vi "Read Write App Config.vi"(7 "Write (F)":bool, 8 "Error IN":errorcluster, 10 "App Config IN":T1={"Location"="", "Profiles Path"=path "", "Current Profile"="", "CA Number"="", "Cycles Completed"=0, "PWM Freq (Hz)"=0.0, "Controller Type:"=enum."Kuhnke", "Inform"="", "Pumps Present"=0, "Stagger Time (ms)"=0, "Tank 1 Fuel"="", "Tank 2 Fuel"="", "Serial Numbers"={"Position 1 SN"="", "Position 2 SN"="", "Poaition 3 SN"="", "Position 4 SN"="", "Position 5 SN"="", "Position 6 SN"=""}, "Constant Data Log"=FALSE, "VoltCtrlRef"="", "TenHzFrequency"=0, "VoltageSelect"=FALSE, "Watlow Present"=FALSE, "Temp 1"=0.0, "Temp 2"=0.0, "V_Run PI?"=FALSE, "Voltage Limits"={"V_Step"=1e-05, "V_CmdMax"=0.0, "V_CmdMin"=0.0}, "Voltage Far PI"={"V_FarSlew"=10.0, "V_FarKp"=0.0, "V_FarKi"=0.0}, "Voltage Mid PI"={"V_MidSlew"=10.0, "V_MidKp"=0.0, "V_MidKi"=0.0}, "Voltage Close PI"={"V_CloseSlew"=10.0, "V_CloseKp"=0.0, "V_CloseKi"=0.0}, "Voltage Scale"={"V_FFm"=0.0, "V_FFb"=0.0}, "Voltage Cutoffs"={"V_MidCutoff"=0.0, "V_CloseCutoff"=0.0}, "Pressure Scale"={"Pres_FFm"=1e-05, "Pres_FFb"=0.0}, "Temp Format"=0, "Temp Tolerance"=0.0}, 11 "Refnum in":T3) -> (0 "Error OUT":errorcluster, 2 "App Config OUT":T1={"Location"="", "Profiles Path"=path "", "Current Profile"="", "CA Number"="", "Cycles Completed"=0, "PWM Freq (Hz)"=0.0, "Controller Type:"=enum."Kuhnke", "Inform"="", "Pumps Present"=0, "Stagger Time (ms)"=0, "Tank 1 Fuel"="", "Tank 2 Fuel"="", "Serial Numbers"={"Position 1 SN"="", "Position 2 SN"="", "Poaition 3 SN"="", "Position 4 SN"="", "Position 5 SN"="", "Position 6 SN"=""}, "Constant Data Log"=FALSE, "VoltCtrlRef"="", "TenHzFrequency"=0, "VoltageSelect"=FALSE, "Watlow Present"=FALSE, "Temp 1"=0.0, "Temp 2"=0.0, "V_Run PI?"=FALSE, "Voltage Limits"={"V_Step"=1e-05, "V_CmdMax"=0.0, "V_CmdMin"=0.0}, "Voltage Far PI"={"V_FarSlew"=10.0, "V_FarKp"=0.0, "V_FarKi"=0.0}, "Voltage Mid PI"={"V_MidSlew"=10.0, "V_MidKp"=0.0, "V_MidKi"=0.0}, "Voltage Close PI"={"V_CloseSlew"=10.0, "V_CloseKp"=0.0, "V_CloseKi"=0.0}, "Voltage Scale"={"V_FFm"=0.0, "V_FFb"=0.0}, "Voltage Cutoffs"={"V_MidCutoff"=0.0, "V_CloseCutoff"=0.0}, "Pressure Scale"={"Pres_FFm"=1e-05, "Pres_FFb"=0.0}, "Temp Format"=0, "Temp Tolerance"=0.0}, 3 "Refnum out":T3)   [LabVIEW 2013]
uses:
  <vilib>/Utility/config.llb/Config Data RefNum.ctl
  Type Defs/App Config.ctl
  Type Defs/Controller Names.ctl
  <vilib>/Utility/config.llb/Write Key (String).vi
  <vilib>/Utility/config.llb/Write Key (Path).vi
  <vilib>/Utility/config.llb/Write Key (U32).vi
  <vilib>/Utility/config.llb/Write Key (Double).vi
  <vilib>/Utility/config.llb/Write Key (I32).vi
  <vilib>/Utility/config.llb/Write Key (Boolean).vi
  <vilib>/Utility/config.llb/Read Key (String).vi
  <vilib>/Utility/config.llb/Read Key (Path).vi
  <vilib>/Utility/config.llb/Read Key (U32).vi
  <vilib>/Utility/config.llb/Read Key (Double).vi
  <vilib>/Utility/config.llb/Read Key (I32).vi
  <vilib>/Utility/config.llb/Read Key (Boolean).vi
  <vilib>/Utility/config.llb/NI_LVConfig.lvlib
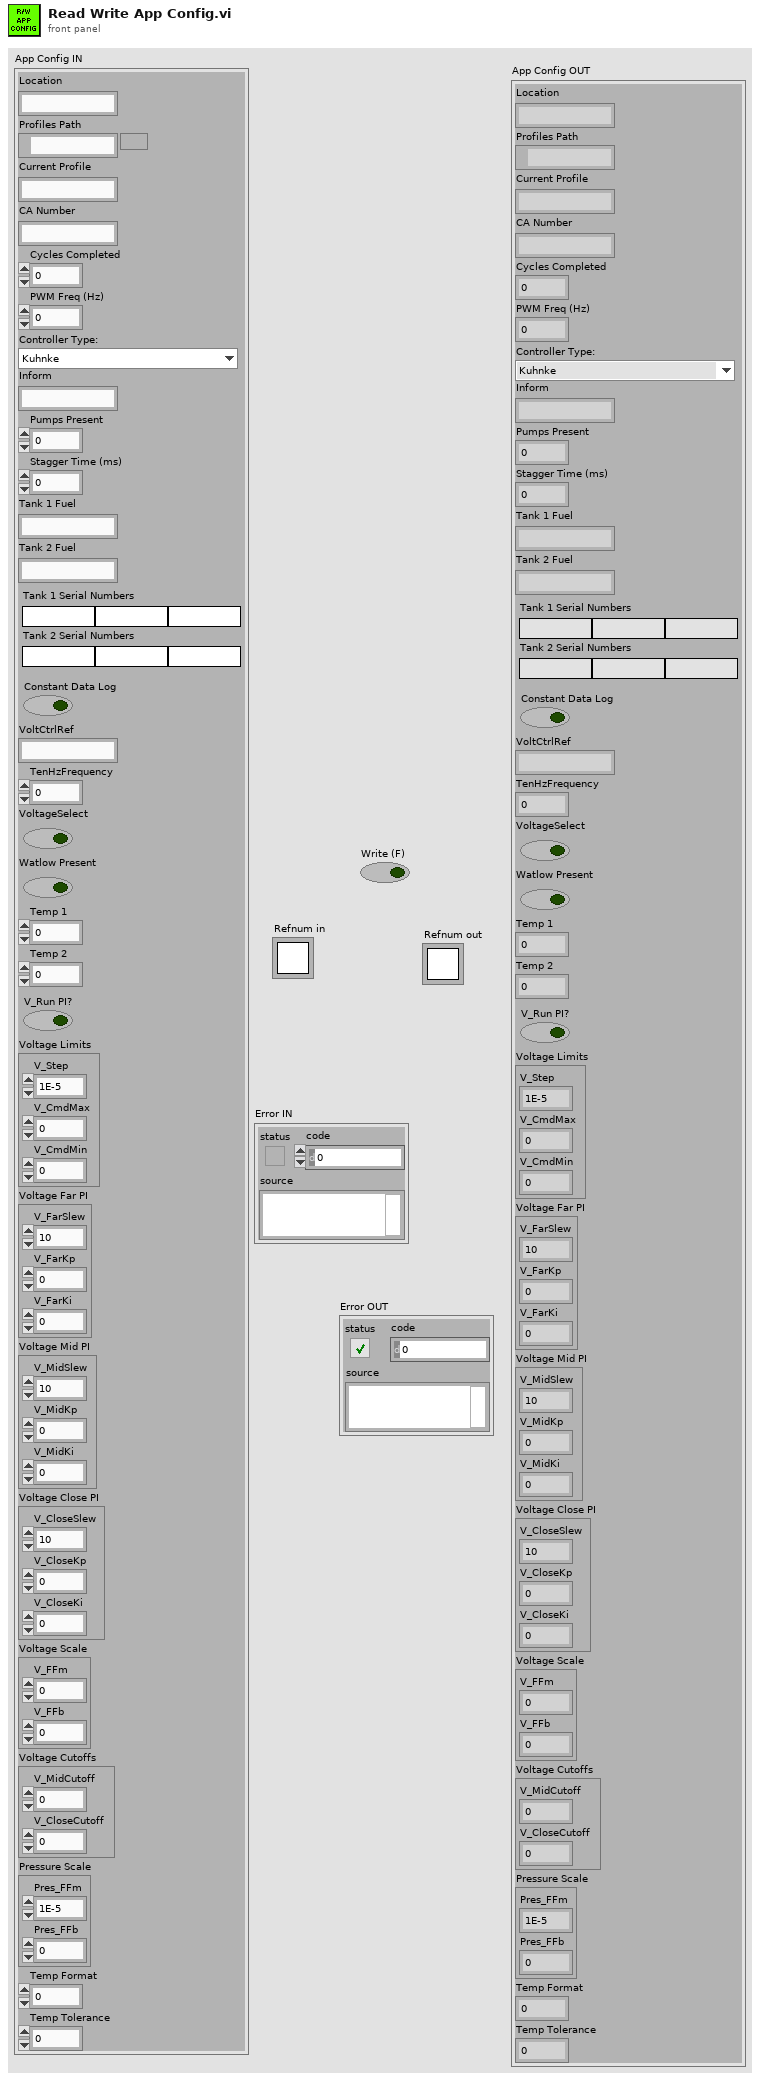
[diagram p1: front panel]
types:
  T1 = typedef "App Config.ctl" = cluster{"Location":string, "Profiles Path":path, "Current Profile":string, "CA Number":string, "Cycles Completed":u32, "PWM Freq (Hz)":dbl, "Controller Type:":T2, "Inform":string, "Pumps Present":u32, "Stagger Time (ms)":i32, "Tank 1 Fuel":string, "Tank 2 Fuel":string, "Serial Numbers":cluster{"Position 1 SN":string, "Position 2 SN":string, "Poaition 3 SN":string, "Position 4 SN":string, "Position 5 SN":string, "Position 6 SN":string}, "Constant Data Log":bool, "VoltCtrlRef":string, "TenHzFrequency":u32, "VoltageSelect":bool, "Watlow Present":bool, "Temp 1":dbl, "Temp 2":dbl, "V_Run PI?":bool, "Voltage Limits":cluster{"V_Step":dbl, "V_CmdMax":dbl, "V_CmdMin":dbl}, "Voltage Far PI":cluster{"V_FarSlew":dbl, "V_FarKp":dbl, "V_FarKi":dbl}, "Voltage Mid PI":cluster{"V_MidSlew":dbl, "V_MidKp":dbl, "V_MidKi":dbl}, "Voltage Close PI":cluster{"V_CloseSlew":dbl, "V_CloseKp":dbl, "V_CloseKi":dbl}, "Voltage Scale":cluster{"V_FFm":dbl, "V_FFb":dbl}, "Voltage Cutoffs":cluster{"V_MidCutoff":dbl, "V_CloseCutoff":dbl}, "Pressure Scale":cluster{"Pres_FFm":dbl, "Pres_FFb":dbl}, "Temp Format":i32, "Temp Tolerance":dbl}
  T2 = typedef "Controller Names.ctl" = enum16{"Kuhnke", "Helbako BLDC", "Conti", "Hella BLDC OL PWM", "Hella BLDC Turbine OL PWM", "Helbako (old)", "TI PWM", "PSA", "Hella Gas", "Hella Diesel", "8 Comm", "10 Comm", "8 Comm Hella", "10 Comm Hella", "8 Comm Omron", "10 Comm Omron", "8 Comm Nissan", "10 Comm Nissan"}
  T3 = typedef "NI_LVConfig.lvlib/Config Data RefNum.ctl" = refnum<k1>
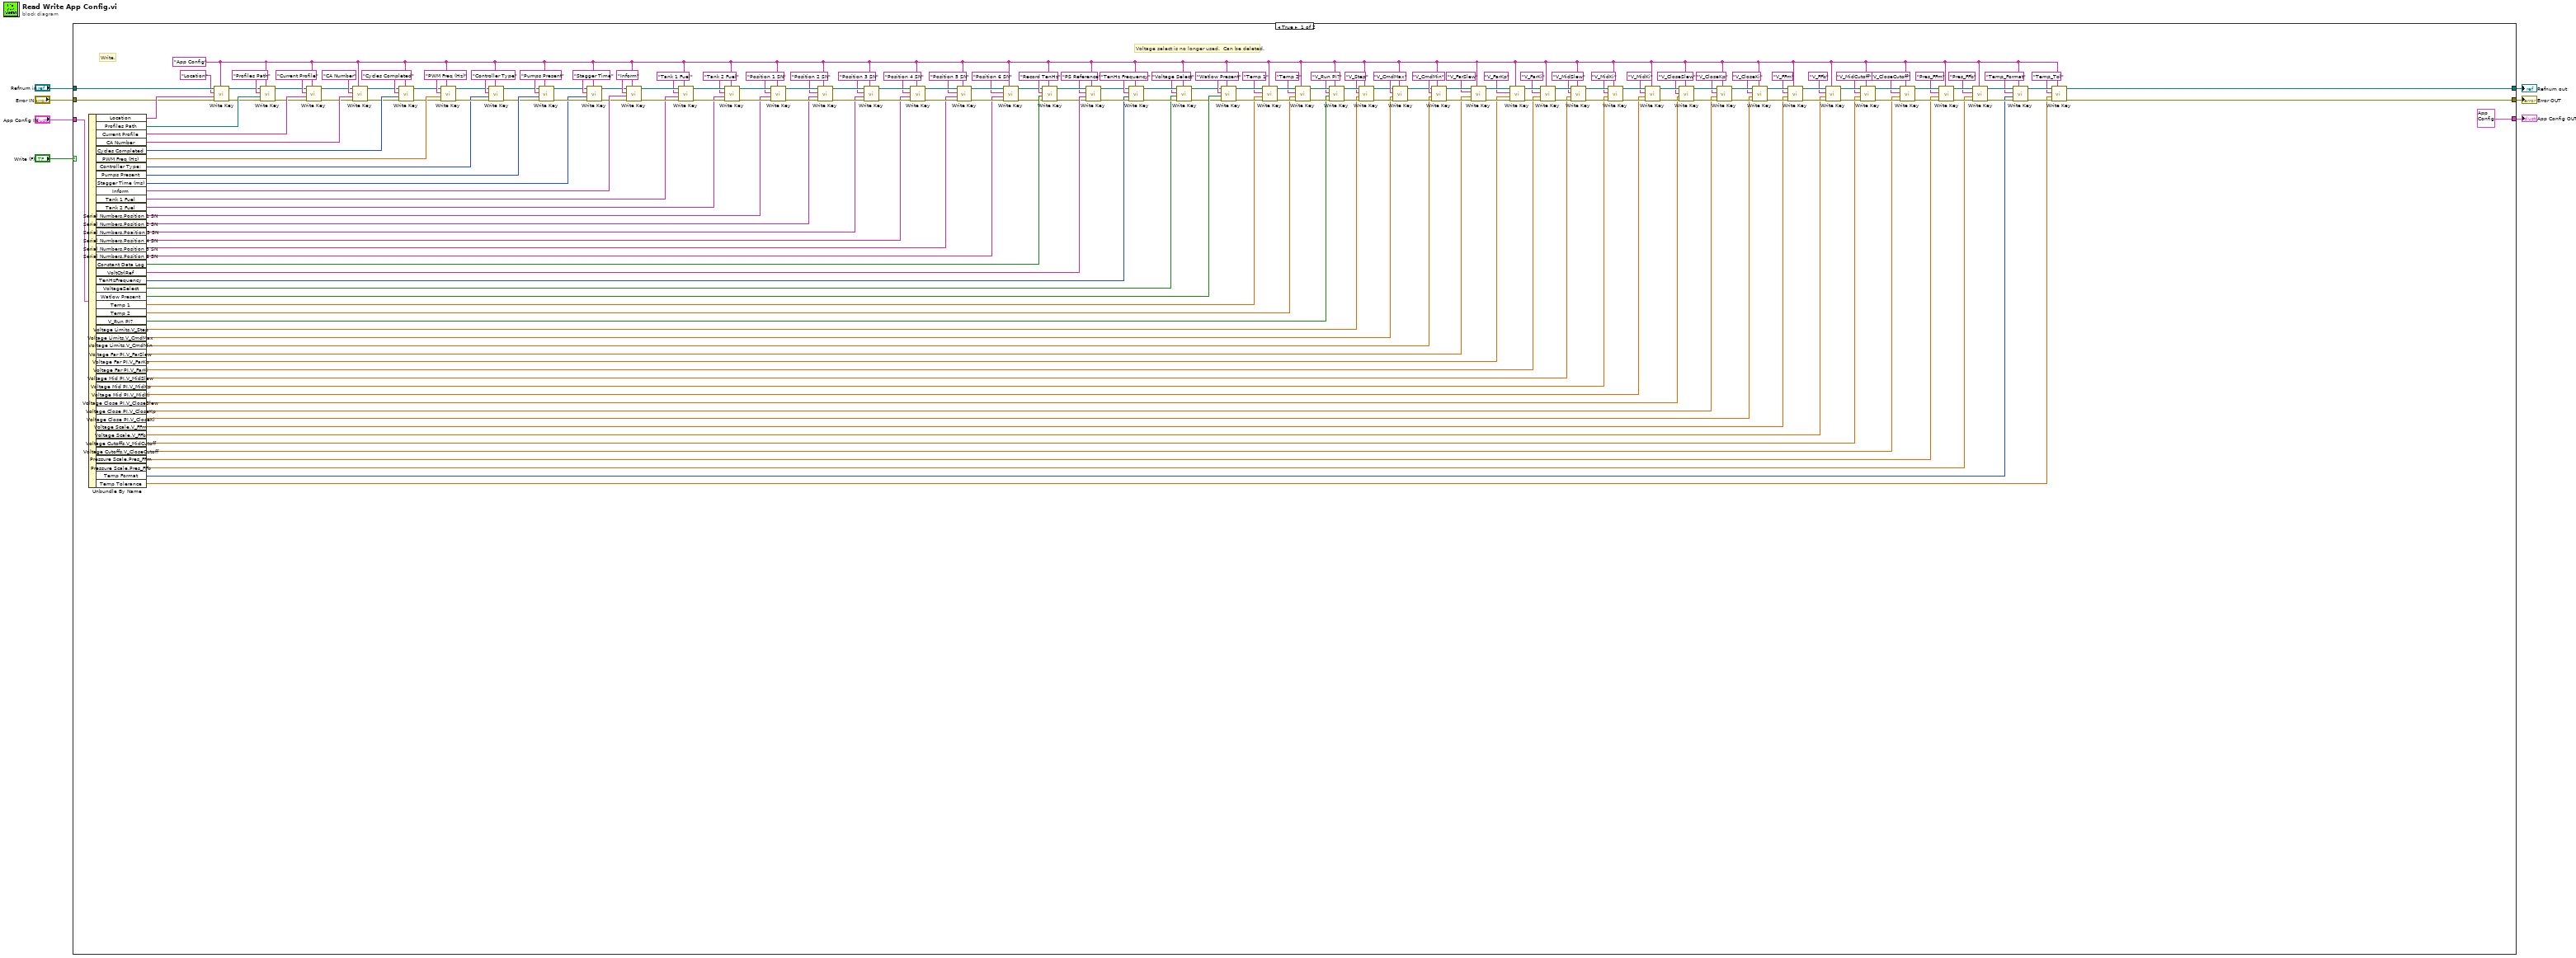
[diagram p0: block diagram]
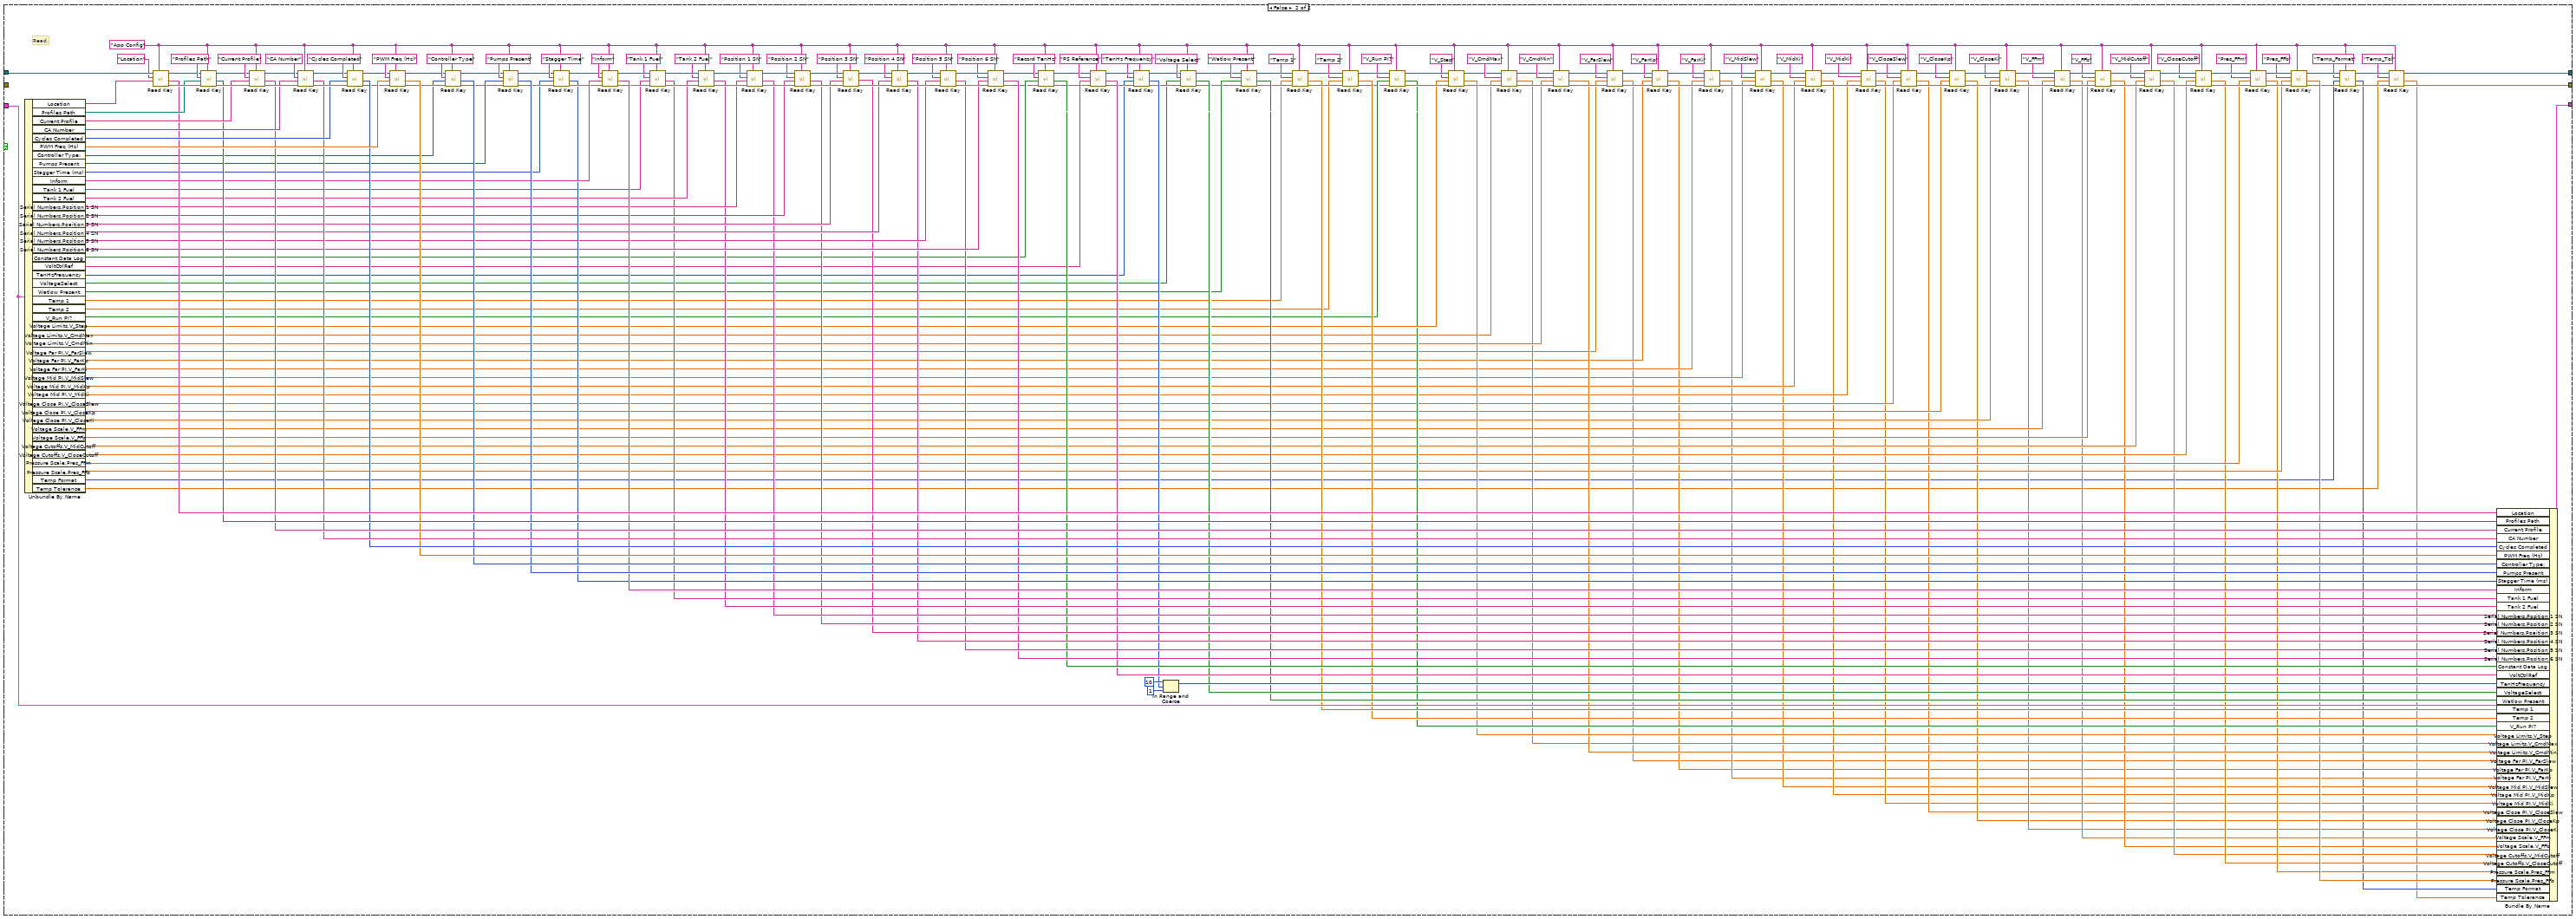
[diagram p2: hidden frame]
diagram:
  n1 = case shown="True" "Write (F)" {
    tunnel: "App Config IN" -> [w196 w385]
    tunnel: "Refnum in" -> [w195 w433]
    tunnel: [w13 w204] -> w4
    tunnel: [w14 w203] -> w3
    tunnel: [T1 {"Location"="", "Profiles Path"=path "", "Current Profile"="", "CA Number"="", "Cycles Completed"=0, "PWM Freq (Hz)"=0.0, "Controller Type:"=enum."Kuhnke", "Inform"="", "Pumps Present"=0, "Stagger Time (ms)"=0, "Tank 1 Fuel"="", "Tank 2 Fuel"="", "Serial Numbers"={"Position 1 SN"="", "Position 2 SN"="", "Poaition 3 SN"="", "Position 4 SN"="", "Position 5 SN"="", "Position 6 SN"=""}, "Constant Data Log"=FALSE, "VoltCtrlRef"="", "TenHzFrequency"=0, "VoltageSelect"=FALSE, "Watlow Present"=FALSE, "Temp 1"=0.0, "Temp 2"=0.0, "V_Run PI?"=FALSE, "Voltage Limits"={"V_Step"=0.0, "V_CmdMax"=0.0, "V_CmdMin"=0.0}, "Voltage Far PI"={"V_FarSlew"=0.0, "V_FarKp"=0.0, "V_FarKi"=0.0}, "Voltage Mid PI"={"V_MidSlew"=0.0, "V_MidKp"=0.0, "V_MidKi"=0.0}, "Voltage Close PI"={"V_CloseSlew"=0.0, "V_CloseKp"=0.0, "V_CloseKi"=0.0}, "Voltage Scale"={"V_FFm"=0.0, "V_FFb"=0.0}, "Voltage Cutoffs"={"V_MidCutoff"=0.0, "V_CloseCutoff"=0.0}, "Pressure Scale"={"Pres_FFm"=0.0, "Pres_FFb"=0.0}, "Temp Format"=0, "Temp Tolerance"=0.0} ("App Config IN") w384] -> w2
    tunnel: "Error IN" -> [w173 _]
    frame True {
      w12 = "App Config" ("section")
      # "Voltage select is no longer used.  Can be deleted."
      # "Write."
      n2 = Unbundle By Name(w196) -> ("Location"=w193:string, "Profiles Path"=w187:path, "Current Profile"=w186:string, "CA Number"=w185:string, "Cycles Completed"=w184:u32, "PWM Freq (Hz)"=w183:dbl, "Controller Type:"=w170:T2, "Pumps Present"=w165:u32, "Stagger Time (ms)"=w155:i32, "Inform"=w161:string, "Tank 1 Fuel"=w138:string, "Tank 2 Fuel"=w137:string, "Serial Numbers.Position 1 SN"=w136:string, "Serial Numbers.Position 2 SN"=w135:string, "Serial Numbers.Poaition 3 SN"=w134:string, "Serial Numbers.Position 4 SN"=w133:string, "Serial Numbers.Position 5 SN"=w132:string, "Serial Numbers.Position 6 SN"=w131:string, "Constant Data Log"=w121:bool, "VoltCtrlRef"=w120:string, "TenHzFrequency"=w113:u32, "VoltageSelect"=w107:bool, "Watlow Present"=w105:bool, "Temp 1"=w95:dbl, "Temp 2"=w96:dbl, "V_Run PI?"=w90:bool, "Voltage Limits.V_Step"=w89:dbl, "Voltage Limits.V_CmdMax"=w72:dbl, "Voltage Limits.V_CmdMin"=w71:dbl, "Voltage Far PI.V_FarSlew"=w33:dbl, "Voltage Far PI.V_FarKp"=w32:dbl, "Voltage Far PI.V_FarKi"=w31:dbl, "Voltage Mid PI.V_MidSlew"=w30:dbl, "Voltage Mid PI.V_MidKp"=w29:dbl, "Voltage Mid PI.V_MidKi"=w28:dbl, "Voltage Close PI.V_CloseSlew"=w27:dbl, "Voltage Close PI.V_CloseKp"=w26:dbl, "Voltage Close PI.V_CloseKi"=w25:dbl, "Voltage Scale.V_FFm"=w24:dbl, "Voltage Scale.V_FFb"=w23:dbl, "Voltage Cutoffs.V_MidCutoff"=w22:dbl, "Voltage Cutoffs.V_CloseCutoff"=w21:dbl, "Pressure Scale.Pres_FFm"=w20:dbl, "Pressure Scale.Pres_FFb"=w19:dbl, "Temp Format"=w9:i32, "Temp Tolerance"=w8:dbl)
      n3 = call-poly <vilib>:"Write Key.vi"("section"=w12, "error in (no error)"=w173, "value"=w193, "key"="Location" ("section"), "refnum"=w195) -> ("error out"=w182:errorcluster, "refnum out"=w181:T3)  [unwired: 4 in, 1 out]
      n4 = call-poly <vilib>:"Write Key.vi"("section"=w12, "error in (no error)"=w182, "value"=w187, "key"="Profiles Path" ("section"), "refnum"=w181) -> ("error out"=w179:errorcluster, "refnum out"=w180:T3)  [unwired: 4 in, 1 out]
      n5 = call-poly <vilib>:"Write Key.vi"("section"=w12, "error in (no error)"=w179, "value"=w186, "key"="Current Profile" ("section"), "refnum"=w180) -> ("error out"=w177:errorcluster, "refnum out"=w178:T3)  [unwired: 4 in, 1 out]
      n6 = call-poly <vilib>:"Write Key.vi"("section"=w12, "error in (no error)"=w177, "value"=w185, "key"="CA Number" ("section"), "refnum"=w178) -> ("error out"=w175:errorcluster, "refnum out"=w176:T3)  [unwired: 4 in, 1 out]
      n7 = call-poly <vilib>:"Write Key.vi"("section"=w12, "error in (no error)"=w175, "value"=w184, "key"="Cycles Completed" ("section"), "refnum"=w176) -> ("error out"=w167:errorcluster, "refnum out"=w168:T3)  [unwired: 4 in, 1 out]
      n8 = call-poly <vilib>:"Write Key.vi"("section"=w12, "error in (no error)"=w167, "value"=w183, "key"="PWM Freq (Hz)" ("section"), "refnum"=w168) -> ("error out"=w171:errorcluster, "refnum out"=w169:T3)  [unwired: 4 in, 1 out]
      n9 = call-poly <vilib>:"Write Key.vi"("section"=w12, "error in (no error)"=w171, "value"=w170, "key"="Controller Type" ("section"), "refnum"=w169) -> ("error out"=w163:errorcluster, "refnum out"=w164:T3)  [unwired: 4 in, 1 out]
      n10 = call-poly <vilib>:"Write Key.vi"("section"=w12, "error in (no error)"=w163, "value"=w165, "key"="Pumps Present" ("section"), "refnum"=w164) -> ("error out"=w158:errorcluster, "refnum out"=w159:T3)  [unwired: 4 in, 1 out]
      n11 = call-poly <vilib>:"Write Key.vi"("section"=w12, "error in (no error)"=w158, "value"=w155, "key"="Stagger Time" ("section"), "refnum"=w159) -> ("error out"=w157:errorcluster, "refnum out"=w156:T3)  [unwired: 4 in, 1 out]
      n12 = call-poly <vilib>:"Write Key.vi"("section"=w12, "error in (no error)"=w157, "value"=w161, "key"="Inform" ("section"), "refnum"=w156) -> ("error out"=w139:errorcluster, "refnum out"=w154:T3)  [unwired: 4 in, 1 out]
      n13 = call-poly <vilib>:"Write Key.vi"("section"=w12, "error in (no error)"=w139, "value"=w138, "key"="Tank 1 Fuel", "refnum"=w154) -> ("error out"=w140:errorcluster, "refnum out"=w153:T3)  [unwired: 4 in, 1 out]
      n14 = call-poly <vilib>:"Write Key.vi"("section"=w12, "error in (no error)"=w140, "value"=w137, "key"="Tank 2 Fuel", "refnum"=w153) -> ("error out"=w141:errorcluster, "refnum out"=w152:T3)  [unwired: 4 in, 1 out]
      n15 = call-poly <vilib>:"Write Key.vi"("section"=w12, "error in (no error)"=w141, "value"=w136, "key"="Position 1 SN", "refnum"=w152) -> ("error out"=w142:errorcluster, "refnum out"=w151:T3)  [unwired: 4 in, 1 out]
      n16 = call-poly <vilib>:"Write Key.vi"("section"=w12, "error in (no error)"=w142, "value"=w135, "key"="Position 2 SN", "refnum"=w151) -> ("error out"=w143:errorcluster, "refnum out"=w150:T3)  [unwired: 4 in, 1 out]
      n17 = call-poly <vilib>:"Write Key.vi"("section"=w12, "error in (no error)"=w143, "value"=w134, "key"="Position 3 SN", "refnum"=w150) -> ("error out"=w144:errorcluster, "refnum out"=w149:T3)  [unwired: 4 in, 1 out]
      n18 = call-poly <vilib>:"Write Key.vi"("section"=w12, "error in (no error)"=w144, "value"=w133, "key"="Position 4 SN", "refnum"=w149) -> ("error out"=w145:errorcluster, "refnum out"=w148:T3)  [unwired: 4 in, 1 out]
      n19 = call-poly <vilib>:"Write Key.vi"("section"=w12, "error in (no error)"=w145, "value"=w132, "key"="Position 5 SN", "refnum"=w148) -> ("error out"=w146:errorcluster, "refnum out"=w147:T3)  [unwired: 4 in, 1 out]
      n20 = call-poly <vilib>:"Write Key.vi"("section"=w12, "error in (no error)"=w146, "value"=w131, "key"="Position 6 SN", "refnum"=w147) -> ("error out"=w111:errorcluster, "refnum out"=w112:T3)  [unwired: 4 in, 1 out]
      n21 = call-poly <vilib>:"Write Key.vi"("section"=w12, "error in (no error)"=w111, "value"=w121, "key"="Record TenHz", "refnum"=w112) -> ("error out"=w119:errorcluster, "refnum out"=w118:T3)  [unwired: 4 in, 1 out]
      n22 = call-poly <vilib>:"Write Key.vi"("section"=w12, "error in (no error)"=w119, "value"=w120, "key"="PS Reference", "refnum"=w118) -> ("error out"=w115:errorcluster, "refnum out"=w114:T3)  [unwired: 4 in, 1 out]
      n23 = call-poly <vilib>:"Write Key.vi"("section"=w12, "error in (no error)"=w115, "value"=w113, "key"="TenHz Frequency", "refnum"=w114) -> ("error out"=w109:errorcluster, "refnum out"=w110:T3)  [unwired: 4 in, 1 out]
      n24 = call-poly <vilib>:"Write Key.vi"("section"=w12, "error in (no error)"=w109, "value"=w107, "key"="Voltage Select", "refnum"=w110) -> ("error out"=w103:errorcluster, "refnum out"=w104:T3)  [unwired: 4 in, 1 out]
      n25 = call-poly <vilib>:"Write Key.vi"("section"=w12, "error in (no error)"=w103, "value"=w105, "key"="Watlow Present", "refnum"=w104) -> ("error out"=w100:errorcluster, "refnum out"=w102:T3)  [unwired: 4 in, 1 out]
      n26 = call-poly <vilib>:"Write Key.vi"("section"=w12, "error in (no error)"=w100, "value"=w95, "key"="Temp 1", "refnum"=w102) -> ("error out"=w99:errorcluster, "refnum out"=w101:T3)  [unwired: 4 in, 1 out]
      n27 = call-poly <vilib>:"Write Key.vi"("section"=w12, "error in (no error)"=w99, "value"=w96, "key"="Temp 2", "refnum"=w101) -> ("error out"=w92:errorcluster, "refnum out"=w93:T3)  [unwired: 4 in, 1 out]
      n28 = call-poly <vilib>:"Write Key.vi"("section"=w12, "error in (no error)"=w92, "value"=w90, "key"="V_Run PI?" ("section"), "refnum"=w93) -> ("error out"=w91:errorcluster, "refnum out"=w94:T3)  [unwired: 4 in, 1 out]
      n29 = call-poly <vilib>:"Write Key.vi"("section"=w12, "error in (no error)"=w91, "value"=w89, "key"="V_Step" ("section"), "refnum"=w94) -> ("error out"=w84:errorcluster, "refnum out"=w78:T3)  [unwired: 4 in, 1 out]
      n30 = call-poly <vilib>:"Write Key.vi"("section"=w12, "error in (no error)"=w84, "value"=w72, "key"="V_CmdMax" ("section"), "refnum"=w78) -> ("error out"=w83:errorcluster, "refnum out"=w77:T3)  [unwired: 4 in, 1 out]
      n31 = call-poly <vilib>:"Write Key.vi"("section"=w12, "error in (no error)"=w83, "value"=w71, "key"="V_CmdMin" ("section"), "refnum"=w77) -> ("error out"=w57:errorcluster, "refnum out"=w66:T3)  [unwired: 4 in, 1 out]
      n32 = call-poly <vilib>:"Write Key.vi"("section"=w12, "error in (no error)"=w57, "value"=w33, "key"="V_FarSlew", "refnum"=w66) -> ("error out"=w58:errorcluster, "refnum out"=w65:T3)  [unwired: 4 in, 1 out]
      n33 = call-poly <vilib>:"Write Key.vi"("section"=w12, "error in (no error)"=w58, "value"=w32, "key"="V_FarKp", "refnum"=w65) -> ("error out"=w59:errorcluster, "refnum out"=w64:T3)  [unwired: 4 in, 1 out]
      n34 = call-poly <vilib>:"Write Key.vi"("section"=w12, "error in (no error)"=w59, "value"=w31, "key"="V_FarKi", "refnum"=w64) -> ("error out"=w60:errorcluster, "refnum out"=w63:T3)  [unwired: 4 in, 1 out]
      n35 = call-poly <vilib>:"Write Key.vi"("section"=w12, "error in (no error)"=w60, "value"=w30, "key"="V_MidSlew", "refnum"=w63) -> ("error out"=w61:errorcluster, "refnum out"=w62:T3)  [unwired: 4 in, 1 out]
      n36 = call-poly <vilib>:"Write Key.vi"("section"=w12, "error in (no error)"=w61, "value"=w29, "key"="V_MidKi", "refnum"=w62) -> ("error out"=w82:errorcluster, "refnum out"=w76:T3)  [unwired: 4 in, 1 out]
      n37 = call-poly <vilib>:"Write Key.vi"("section"=w12, "error in (no error)"=w82, "value"=w28, "key"="V_MidKi", "refnum"=w76) -> ("error out"=w81:errorcluster, "refnum out"=w75:T3)  [unwired: 4 in, 1 out]
      n38 = call-poly <vilib>:"Write Key.vi"("section"=w12, "error in (no error)"=w81, "value"=w27, "key"="V_CloseSlew", "refnum"=w75) -> ("error out"=w80:errorcluster, "refnum out"=w74:T3)  [unwired: 4 in, 1 out]
      n39 = call-poly <vilib>:"Write Key.vi"("section"=w12, "error in (no error)"=w80, "value"=w26, "key"="V_CloseKp", "refnum"=w74) -> ("error out"=w79:errorcluster, "refnum out"=w73:T3)  [unwired: 4 in, 1 out]
      n40 = call-poly <vilib>:"Write Key.vi"("section"=w12, "error in (no error)"=w79, "value"=w25, "key"="V_CloseKi", "refnum"=w73) -> ("error out"=w67:errorcluster, "refnum out"=w70:T3)  [unwired: 4 in, 1 out]
      n41 = call-poly <vilib>:"Write Key.vi"("section"=w12, "error in (no error)"=w67, "value"=w24, "key"="V_FFm", "refnum"=w70) -> ("error out"=w68:errorcluster, "refnum out"=w69:T3)  [unwired: 4 in, 1 out]
      n42 = call-poly <vilib>:"Write Key.vi"("section"=w12, "error in (no error)"=w68, "value"=w23, "key"="V_FFb", "refnum"=w69) -> ("error out"=w49:errorcluster, "refnum out"=w53:T3)  [unwired: 4 in, 1 out]
      n43 = call-poly <vilib>:"Write Key.vi"("section"=w12, "error in (no error)"=w49, "value"=w22, "key"="V_MidCutoff", "refnum"=w53) -> ("error out"=w50:errorcluster, "refnum out"=w54:T3)  [unwired: 4 in, 1 out]
      n44 = call-poly <vilib>:"Write Key.vi"("section"=w12, "error in (no error)"=w50, "value"=w21, "key"="V_CloseCutoff", "refnum"=w54) -> ("error out"=w51:errorcluster, "refnum out"=w55:T3)  [unwired: 4 in, 1 out]
      n45 = call-poly <vilib>:"Write Key.vi"("section"=w12, "error in (no error)"=w51, "value"=w20, "key"="Pres_FFm", "refnum"=w55) -> ("error out"=w52:errorcluster, "refnum out"=w56:T3)  [unwired: 4 in, 1 out]
      n46 = call-poly <vilib>:"Write Key.vi"("section"=w12, "error in (no error)"=w52, "value"=w19, "key"="Pres_FFb", "refnum"=w56) -> ("error out"=w15:errorcluster, "refnum out"=w18:T3)  [unwired: 4 in, 1 out]
      n47 = call-poly <vilib>:"Write Key.vi"("section"=w12, "error in (no error)"=w15, "value"=w9, "key"="Temp_Format", "refnum"=w18) -> ("error out"=w16:errorcluster, "refnum out"=w17:T3)  [unwired: 4 in, 1 out]
      n48 = call-poly <vilib>:"Write Key.vi"("section"=w12, "error in (no error)"=w16, "value"=w8, "key"="Temp_Tol", "refnum"=w17) -> ("error out"=w14:errorcluster, "refnum out"=w13:T3)  [unwired: 4 in, 1 out]
    }
    frame False {
      w209 = "App Config" ("section")
      # "Read."
      n49 = Unbundle By Name(w385) -> ("Location"=w418:string, "Profiles Path"=w417:path, "Current Profile"=w416:string, "CA Number"=w415:string, "Cycles Completed"=w414:u32, "PWM Freq (Hz)"=w413:dbl, "Controller Type:"=w331:T2, "Pumps Present"=w399:u32, "Stagger Time (ms)"=w387:i32, "Inform"=w394:string, "Tank 1 Fuel"=w359:string, "Tank 2 Fuel"=w358:string, "Serial Numbers.Position 1 SN"=w357:string, "Serial Numbers.Position 2 SN"=w356:string, "Serial Numbers.Poaition 3 SN"=w355:string, "Serial Numbers.Position 4 SN"=w354:string, "Serial Numbers.Position 5 SN"=w353:string, "Serial Numbers.Position 6 SN"=w352:string, "Constant Data Log"=w342:bool, "VoltCtrlRef"=w339:string, "TenHzFrequency"=w333:u32, "VoltageSelect"=w321:bool, "Watlow Present"=w318:bool, "Temp 1"=w306:dbl, "Temp 2"=w305:dbl, "V_Run PI?"=w302:bool, "Voltage Limits.V_Step"=w301:dbl, "Voltage Limits.V_CmdMax"=w278:dbl, "Voltage Limits.V_CmdMin"=w277:dbl, "Voltage Far PI.V_FarSlew"=w239:dbl, "Voltage Far PI.V_FarKp"=w238:dbl, "Voltage Far PI.V_FarKi"=w237:dbl, "Voltage Mid PI.V_MidSlew"=w236:dbl, "Voltage Mid PI.V_MidKp"=w235:dbl, "Voltage Mid PI.V_MidKi"=w234:dbl, "Voltage Close PI.V_CloseSlew"=w233:dbl, "Voltage Close PI.V_CloseKp"=w232:dbl, "Voltage Close PI.V_CloseKi"=w231:dbl, "Voltage Scale.V_FFm"=w230:dbl, "Voltage Scale.V_FFb"=w229:dbl, "Voltage Cutoffs.V_MidCutoff"=w228:dbl, "Voltage Cutoffs.V_CloseCutoff"=w227:dbl, "Pressure Scale.Pres_FFm"=w226:dbl, "Pressure Scale.Pres_FFb"=w225:dbl, "Temp Format"=w197:i32, "Temp Tolerance"=w198:dbl)
      n50 = call-poly <vilib>:"Read Key.vi"("section"=w209, "default value"=w418, "key"="Location" ("section"), "refnum"=w433) -> ("error out"=w426:errorcluster, "value"=w412:string, "refnum out"=w425:T3)  [unwired: 4 in, 1 out]
      n51 = call-poly <vilib>:"Read Key.vi"("section"=w209, "error in (no error)"=w426, "default value"=w417, "key"="Profiles Path" ("section"), "refnum"=w425) -> ("error out"=w423:errorcluster, "value"=w411:path, "refnum out"=w424:T3)  [unwired: 3 in, 1 out]
      n52 = call-poly <vilib>:"Read Key.vi"("section"=w209, "error in (no error)"=w423, "default value"=w416, "key"="Current Profile" ("section"), "refnum"=w424) -> ("error out"=w421:errorcluster, "value"=w410:string, "refnum out"=w422:T3)  [unwired: 3 in, 1 out]
      n53 = call-poly <vilib>:"Read Key.vi"("section"=w209, "error in (no error)"=w421, "default value"=w415, "key"="CA Number" ("section"), "refnum"=w422) -> ("error out"=w419:errorcluster, "value"=w409:string, "refnum out"=w420:T3)  [unwired: 3 in, 1 out]
      n54 = call-poly <vilib>:"Read Key.vi"("section"=w209, "error in (no error)"=w419, "default value"=w414, "key"="Cycles Completed" ("section"), "refnum"=w420) -> ("error out"=w401:errorcluster, "value"=w408:u32, "refnum out"=w402:T3)  [unwired: 3 in, 1 out]
      n55 = call-poly <vilib>:"Read Key.vi"("section"=w209, "error in (no error)"=w401, "default value"=w413, "key"="PWM Freq (Hz)" ("section"), "refnum"=w402) -> ("error out"=w404:errorcluster, "value"=w407:dbl, "refnum out"=w405:T3)  [unwired: 3 in, 1 out]
      n56 = call-poly <vilib>:"Read Key.vi"("section"=w209, "error in (no error)"=w404, "default value"=w331, "key"="Controller Type" ("section"), "refnum"=w405) -> ("error out"=w398:errorcluster, "value"=w403:i32, "refnum out"=w397:T3)  [unwired: 3 in, 1 out]
      n57 = call-poly <vilib>:"Read Key.vi"("section"=w209, "error in (no error)"=w398, "default value"=w399, "key"="Pumps Present" ("section"), "refnum"=w397) -> ("error out"=w391:errorcluster, "value"=w396:u32, "refnum out"=w390:T3)  [unwired: 3 in, 1 out]
      n58 = call-poly <vilib>:"Read Key.vi"("section"=w209, "error in (no error)"=w391, "default value"=w387, "key"="Stagger Time" ("section"), "refnum"=w390) -> ("error out"=w388:errorcluster, "value"=w386:i32, "refnum out"=w389:T3)  [unwired: 3 in, 1 out]
      n59 = call-poly <vilib>:"Read Key.vi"("section"=w209, "error in (no error)"=w388, "default value"=w394, "key"="Inform" ("section"), "refnum"=w389) -> ("error out"=w375:errorcluster, "value"=w393:string, "refnum out"=w383:T3)  [unwired: 3 in, 1 out]
      n60 = call-poly <vilib>:"Read Key.vi"("section"=w209, "error in (no error)"=w375, "default value"=w359, "key"="Tank 1 Fuel", "refnum"=w383) -> ("error out"=w374:errorcluster, "value"=w351:string, "refnum out"=w382:T3)  [unwired: 3 in, 1 out]
      n61 = call-poly <vilib>:"Read Key.vi"("section"=w209, "error in (no error)"=w374, "default value"=w358, "key"="Tank 2 Fuel", "refnum"=w382) -> ("error out"=w373:errorcluster, "value"=w350:string, "refnum out"=w381:T3)  [unwired: 3 in, 1 out]
      n62 = call-poly <vilib>:"Read Key.vi"("section"=w209, "error in (no error)"=w373, "default value"=w357, "key"="Position 1 SN", "refnum"=w381) -> ("error out"=w372:errorcluster, "value"=w349:string, "refnum out"=w380:T3)  [unwired: 3 in, 1 out]
      n63 = call-poly <vilib>:"Read Key.vi"("section"=w209, "error in (no error)"=w372, "default value"=w356, "key"="Position 2 SN", "refnum"=w380) -> ("error out"=w371:errorcluster, "value"=w348:string, "refnum out"=w379:T3)  [unwired: 3 in, 1 out]
      n64 = call-poly <vilib>:"Read Key.vi"("section"=w209, "error in (no error)"=w371, "default value"=w355, "key"="Position 3 SN", "refnum"=w379) -> ("error out"=w370:errorcluster, "value"=w347:string, "refnum out"=w378:T3)  [unwired: 3 in, 1 out]
      n65 = call-poly <vilib>:"Read Key.vi"("section"=w209, "error in (no error)"=w370, "default value"=w354, "key"="Position 4 SN", "refnum"=w378) -> ("error out"=w369:errorcluster, "value"=w346:string, "refnum out"=w377:T3)  [unwired: 3 in, 1 out]
      n66 = call-poly <vilib>:"Read Key.vi"("section"=w209, "error in (no error)"=w369, "default value"=w353, "key"="Position 5 SN", "refnum"=w377) -> ("error out"=w368:errorcluster, "value"=w345:string, "refnum out"=w376:T3)  [unwired: 3 in, 1 out]
      n67 = call-poly <vilib>:"Read Key.vi"("section"=w209, "error in (no error)"=w368, "default value"=w352, "key"="Position 6 SN", "refnum"=w376) -> ("error out"=w325:errorcluster, "value"=w344:string, "refnum out"=w326:T3)  [unwired: 3 in, 1 out]
      n68 = call-poly <vilib>:"Read Key.vi"("section"=w209, "error in (no error)"=w325, "default value"=w342, "key"="Record TenHz", "refnum"=w326) -> ("error out"=w338:errorcluster, "value"=w341:bool, "refnum out"=w337:T3)  [unwired: 3 in, 1 out]
      n69 = call-poly <vilib>:"Read Key.vi"("section"=w209, "error in (no error)"=w338, "default value"=w339, "key"="PS Reference", "refnum"=w337) -> ("error out"=w334:errorcluster, "value"=w336:string, "refnum out"=w335:T3)  [unwired: 3 in, 1 out]
      n70 = call-poly <vilib>:"Read Key.vi"("section"=w209, "error in (no error)"=w334, "default value"=w333, "key"="TenHz Frequency", "refnum"=w335) -> ("error out"=w322:errorcluster, "value"=w328:u32, "refnum out"=w323:T3)  [unwired: 3 in, 1 out]
      n71 = In Range and Coerce(upper limit=u32 10, x=w328, lower limit=u32 1) -> (coerced(x)=w327:u32)  [unwired: 1 out]
      n72 = call-poly <vilib>:"Read Key.vi"("section"=w209, "error in (no error)"=w322, "default value"=w321, "key"="Voltage Select", "refnum"=w323) -> ("error out"=w315:errorcluster, "value"=w320:bool, "refnum out"=w316:T3)  [unwired: 3 in, 1 out]
      n73 = call-poly <vilib>:"Read Key.vi"("section"=w209, "error in (no error)"=w315, "default value"=w318, "key"="Watlow Present", "refnum"=w316) -> ("error out"=w312:errorcluster, "value"=w317:bool, "refnum out"=w314:T3)  [unwired: 3 in, 1 out]
      n74 = call-poly <vilib>:"Read Key.vi"("section"=w209, "error in (no error)"=w312, "default value"=w306, "key"="Temp 1", "refnum"=w314) -> ("error out"=w311:errorcluster, "value"=w308:dbl, "refnum out"=w313:T3)  [unwired: 3 in, 1 out]
      n75 = call-poly <vilib>:"Read Key.vi"("section"=w209, "error in (no error)"=w311, "default value"=w305, "key"="Temp 2", "refnum"=w313) -> ("error out"=w299:errorcluster, "value"=w307:dbl, "refnum out"=w300:T3)  [unwired: 3 in, 1 out]
      n76 = call-poly <vilib>:"Read Key.vi"("section"=w209, "error in (no error)"=w299, "default value"=w302, "key"="V_Run PI?" ("section"), "refnum"=w300) -> ("error out"=w304:errorcluster, "value"=w298:bool, "refnum out"=w303:T3)  [unwired: 3 in, 1 out]
      n77 = call-poly <vilib>:"Read Key.vi"("section"=w209, "error in (no error)"=w304, "default value"=w301, "key"="V_Step" ("section"), "refnum"=w303) -> ("error out"=w279:errorcluster, "value"=w297:dbl, "refnum out"=w292:T3)  [unwired: 3 in, 1 out]
      n78 = call-poly <vilib>:"Read Key.vi"("section"=w209, "error in (no error)"=w279, "default value"=w278, "key"="V_CmdMax" ("section"), "refnum"=w292) -> ("error out"=w280:errorcluster, "value"=w275:dbl, "refnum out"=w291:T3)  [unwired: 3 in, 1 out]
      n79 = call-poly <vilib>:"Read Key.vi"("section"=w209, "error in (no error)"=w280, "default value"=w277, "key"="V_CmdMin" ("section"), "refnum"=w291) -> ("error out"=w281:errorcluster, "value"=w276:dbl, "refnum out"=w290:T3)  [unwired: 3 in, 1 out]
      n80 = call-poly <vilib>:"Read Key.vi"("section"=w209, "error in (no error)"=w281, "default value"=w239, "key"="V_FarSlew", "refnum"=w290) -> ("error out"=w282:errorcluster, "value"=w210:dbl, "refnum out"=w289:T3)  [unwired: 3 in, 1 out]
      n81 = call-poly <vilib>:"Read Key.vi"("section"=w209, "error in (no error)"=w282, "default value"=w238, "key"="V_FarKp", "refnum"=w289) -> ("error out"=w283:errorcluster, "value"=w211:dbl, "refnum out"=w288:T3)  [unwired: 3 in, 1 out]
      n82 = call-poly <vilib>:"Read Key.vi"("section"=w209, "error in (no error)"=w283, "default value"=w237, "key"="V_FarKi", "refnum"=w288) -> ("error out"=w284:errorcluster, "value"=w212:dbl, "refnum out"=w287:T3)  [unwired: 3 in, 1 out]
      n83 = call-poly <vilib>:"Read Key.vi"("section"=w209, "error in (no error)"=w284, "default value"=w236, "key"="V_MidSlew", "refnum"=w287) -> ("error out"=w285:errorcluster, "value"=w213:dbl, "refnum out"=w286:T3)  [unwired: 3 in, 1 out]
      n84 = call-poly <vilib>:"Read Key.vi"("section"=w209, "error in (no error)"=w285, "default value"=w235, "key"="V_MidKi", "refnum"=w286) -> ("error out"=w274:errorcluster, "value"=w214:dbl, "refnum out"=w271:T3)  [unwired: 3 in, 1 out]
      n85 = call-poly <vilib>:"Read Key.vi"("section"=w209, "error in (no error)"=w274, "default value"=w234, "key"="V_MidKi", "refnum"=w271) -> ("error out"=w273:errorcluster, "value"=w215:dbl, "refnum out"=w272:T3)  [unwired: 3 in, 1 out]
      n86 = call-poly <vilib>:"Read Key.vi"("section"=w209, "error in (no error)"=w273, "default value"=w233, "key"="V_CloseSlew", "refnum"=w272) -> ("error out"=w263:errorcluster, "value"=w216:dbl, "refnum out"=w270:T3)  [unwired: 3 in, 1 out]
      n87 = call-poly <vilib>:"Read Key.vi"("section"=w209, "error in (no error)"=w263, "default value"=w232, "key"="V_CloseKp", "refnum"=w270) -> ("error out"=w264:errorcluster, "value"=w217:dbl, "refnum out"=w269:T3)  [unwired: 3 in, 1 out]
      n88 = call-poly <vilib>:"Read Key.vi"("section"=w209, "error in (no error)"=w264, "default value"=w231, "key"="V_CloseKi", "refnum"=w269) -> ("error out"=w265:errorcluster, "value"=w218:dbl, "refnum out"=w268:T3)  [unwired: 3 in, 1 out]
      n89 = call-poly <vilib>:"Read Key.vi"("section"=w209, "error in (no error)"=w265, "default value"=w230, "key"="V_FFm", "refnum"=w268) -> ("error out"=w266:errorcluster, "value"=w219:dbl, "refnum out"=w267:T3)  [unwired: 3 in, 1 out]
      n90 = call-poly <vilib>:"Read Key.vi"("section"=w209, "error in (no error)"=w266, "default value"=w229, "key"="V_FFb", "refnum"=w267) -> ("error out"=w258:errorcluster, "value"=w220:dbl, "refnum out"=w262:T3)  [unwired: 3 in, 1 out]
      n91 = call-poly <vilib>:"Read Key.vi"("section"=w209, "error in (no error)"=w258, "default value"=w228, "key"="V_MidCutoff", "refnum"=w262) -> ("error out"=w257:errorcluster, "value"=w221:dbl, "refnum out"=w261:T3)  [unwired: 3 in, 1 out]
      n92 = call-poly <vilib>:"Read Key.vi"("section"=w209, "error in (no error)"=w257, "default value"=w227, "key"="V_CloseCutoff", "refnum"=w261) -> ("error out"=w256:errorcluster, "value"=w222:dbl, "refnum out"=w260:T3)  [unwired: 3 in, 1 out]
      n93 = call-poly <vilib>:"Read Key.vi"("section"=w209, "error in (no error)"=w256, "default value"=w226, "key"="Pres_FFm", "refnum"=w260) -> ("error out"=w255:errorcluster, "value"=w223:dbl, "refnum out"=w259:T3)  [unwired: 3 in, 1 out]
      n94 = call-poly <vilib>:"Read Key.vi"("section"=w209, "error in (no error)"=w255, "default value"=w225, "key"="Pres_FFb", "refnum"=w259) -> ("error out"=w208:errorcluster, "value"=w224:dbl, "refnum out"=w206:T3)  [unwired: 3 in, 1 out]
      n95 = call-poly <vilib>:"Read Key.vi"("section"=w209, "error in (no error)"=w208, "default value"=w197, "key"="Temp_Format", "refnum"=w206) -> ("error out"=w207:errorcluster, "value"=w200:i32, "refnum out"=w205:T3)  [unwired: 3 in, 1 out]
      n96 = call-poly <vilib>:"Read Key.vi"("section"=w209, "error in (no error)"=w207, "default value"=w198, "key"="Temp_Tol", "refnum"=w205) -> ("error out"=w203:errorcluster, "value"=w199:dbl, "refnum out"=w204:T3)  [unwired: 3 in, 1 out]
      n97 = Bundle By Name(cluster=w385, "Location"=w412, "Profiles Path"=w411, "Current Profile"=w410, "CA Number"=w409, "Cycles Completed"=w408, "PWM Freq (Hz)"=w407, "Controller Type:"=w403, "Pumps Present"=w396, "Stagger Time (ms)"=w386, "Inform"=w393, "Tank 1 Fuel"=w351, "Tank 2 Fuel"=w350, "Serial Numbers.Position 1 SN"=w349, "Serial Numbers.Position 2 SN"=w348, "Serial Numbers.Poaition 3 SN"=w347, "Serial Numbers.Position 4 SN"=w346, "Serial Numbers.Position 5 SN"=w345, "Serial Numbers.Position 6 SN"=w344, "Constant Data Log"=w341, "VoltCtrlRef"=w336, "TenHzFrequency"=w327, "VoltageSelect"=w320, "Watlow Present"=w317, "Temp 1"=w308, "Temp 2"=w307, "V_Run PI?"=w298, "Voltage Limits.V_Step"=w297, "Voltage Limits.V_CmdMax"=w275, "Voltage Limits.V_CmdMin"=w276, "Voltage Far PI.V_FarSlew"=w210, "Voltage Far PI.V_FarKp"=w211, "Voltage Far PI.V_FarKi"=w212, "Voltage Mid PI.V_MidSlew"=w213, "Voltage Mid PI.V_MidKp"=w214, "Voltage Mid PI.V_MidKi"=w215, "Voltage Close PI.V_CloseSlew"=w216, "Voltage Close PI.V_CloseKp"=w217, "Voltage Close PI.V_CloseKi"=w218, "Voltage Scale.V_FFm"=w219, "Voltage Scale.V_FFb"=w220, "Voltage Cutoffs.V_MidCutoff"=w221, "Voltage Cutoffs.V_CloseCutoff"=w222, "Pressure Scale.Pres_FFm"=w223, "Pressure Scale.Pres_FFb"=w224, "Temp Format"=w200, "Temp Tolerance"=w199) -> (w384:T1)
    }
  }
  "Error OUT" <- w3
  "Refnum out" <- w4
  "App Config OUT" <- w2
